vi "Tag Settings Session.vi"(7 "Database Connection":refnum<k7>, 8 "Error In":errorcluster, 10 "DeviceName":string, 11 "Type":enum16{"Set Settings", "Get Settings"}(ring)=enum."Get Settings") -> (0 "Error Out":errorcluster, 3 "Tag Settings":T1(array[cluster]) {"Vmax" min=-10.0 max=10.0 step=1.0; "Vmin" min=-10.0 max=10.0 step=1.0})   [LabVIEW 2019]
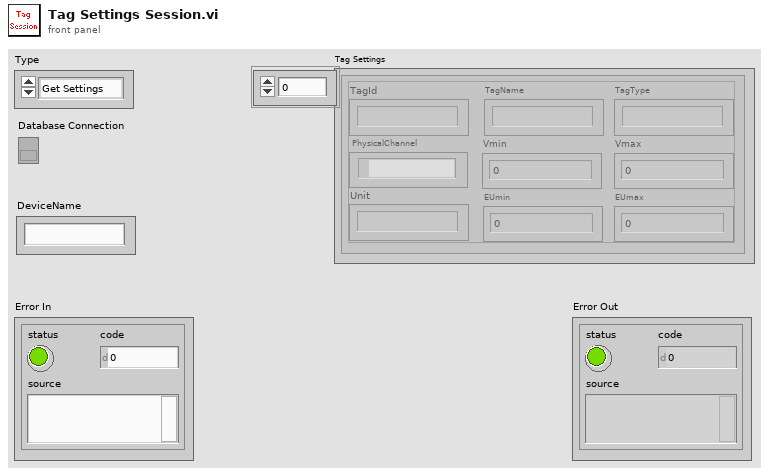
[diagram p1: front panel]
types:
  T1 = cluster{"TagId":string, "TagName":string, "TagType":string, "PhysicalChannel":tag, "Vmin":dbl, "Vmax":dbl, "Unit":string, "EUmin":dbl, "EUmax":dbl}[]
  T2 = cluster{"TagId":string, "TagName":string, "TagType":string, "PhysicalChannel":tag, "Vmin":dbl, "Vmax":dbl, "Unit":string, "EUmin":dbl, "EUmax":dbl}
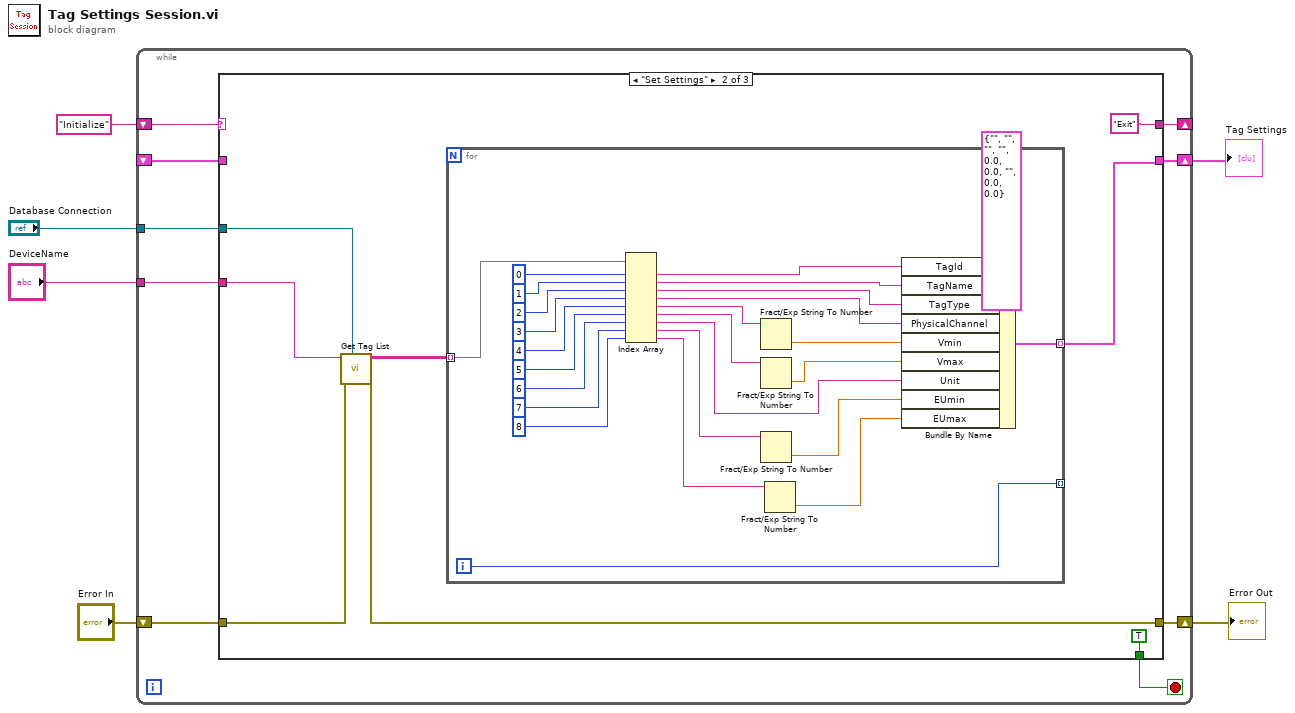
[diagram p0: block diagram]
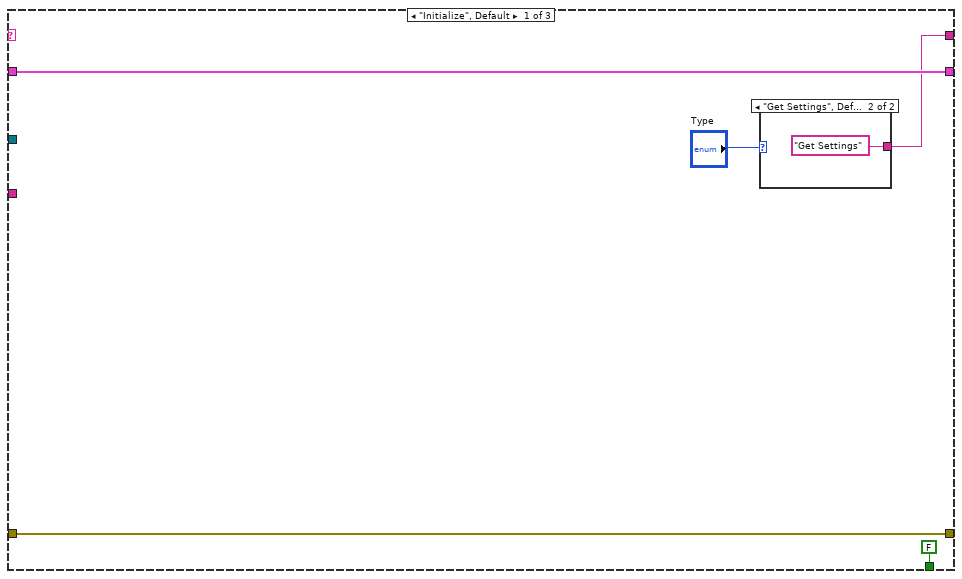
[diagram p2: hidden frame]
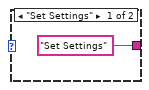
[diagram p3: hidden frame]
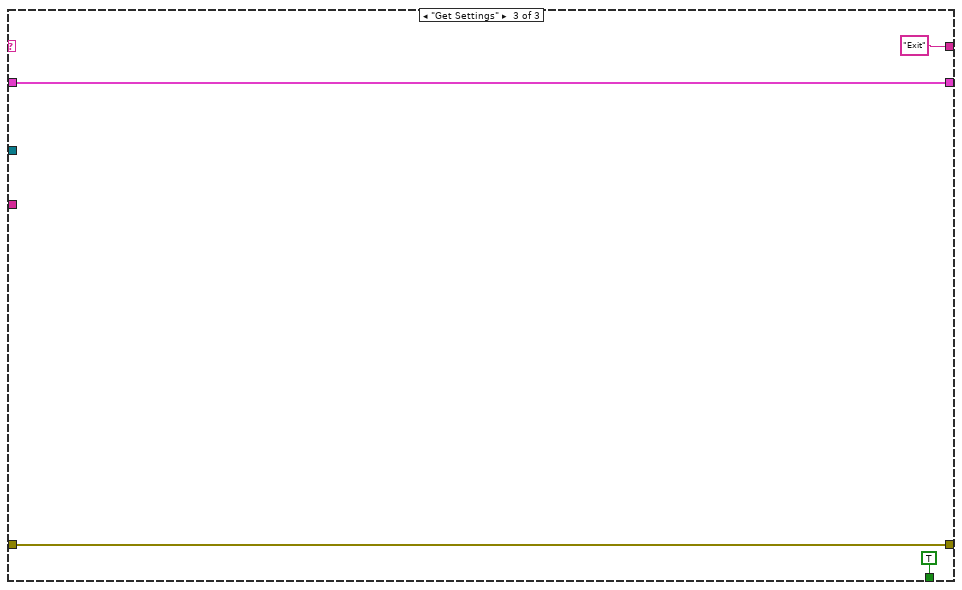
[diagram p4: hidden frame]
diagram:
  n1 = while {
    shift-right: [w10] -> _
    shift-left: "Initialize" ("key") -> [w15]
    shift-right: [w11] -> w3
    shift-left: _ -> [w14]
    shift-right: [w12] -> w4
    shift-left: "Error In" -> [w13]
    tunnel: "Database Connection" -> [w8]
    tunnel: "DeviceName" -> [w7]
    stop <- w9 stop-if-true
    n2 = case shown="\"Set Settings\"" w15 {
      tunnel: w14 -> [w18 _ w57]
      tunnel: w13 -> [w19 w28 w58]
      tunnel: [w19 w27 w58] -> w12
      tunnel: [w18 w23 w57] -> w11
      tunnel: [w16 "Exit" ("key") "Exit" ("key")] -> w10
      tunnel: [FALSE TRUE TRUE] -> w9
      tunnel: w8 -> [_ w26 _]
      tunnel: w7 -> [_ w25 _]
      frame "Initialize", Default {
        n3 = case shown="\"Get Settings\", Default" "Type" {
          tunnel: ["Set Settings" ("key") "Get Settings" ("key")] -> w16
          frame "Set Settings" {
          }
          frame "Get Settings", Default {
          }
        }
      }
      frame "Set Settings" {
        n4 = call "Get Tag List.vi"("Database Connection"=w26, "Error In"=w28, "DeviceName"=w25) -> ("Error Out"=w27:errorcluster, "Tag List"=w24:string[][])  [unwired: 7 in]
        n5 = for {
          tunnel: w24 -> [w55] mode=indexing
          tunnel: [w56] -> w23 mode=indexing
          tunnel: [w31] -> _ mode=indexing
          i -> [w31]
          n6 = Index Array(array=w55, index #1=0 ("index"), index #2=1 ("index"), index #3=2 ("index"), index #4=3 ("index"), index #5=4 ("index"), index #6=5 ("index"), index #7=6 ("index"), index #8=7 ("index"), index #9=8 ("index")) -> (element #1=w53:string, element #2=w44:string, element #3=w43:string, element #4=w42:string, element #5=w41:string, element #6=w38:string, element #7=w37:string, element #8=w36:string, element #9=w34:string)
          n7 = Fract/Exp String To Number(string=w41) -> (number=w40:dbl)  [unwired: 3 in, 1 out]
          n8 = Fract/Exp String To Number(string=w38) -> (number=w39:dbl)  [unwired: 3 in, 1 out]
          n9 = Fract/Exp String To Number(string=w36) -> (number=w35:dbl)  [unwired: 3 in, 1 out]
          n10 = Fract/Exp String To Number(string=w34) -> (number=w33:dbl)  [unwired: 3 in, 1 out]
          n11 = Bundle By Name(cluster=T2 {"TagId"="", "TagName"="", "TagType"="", "PhysicalChannel"="", "Vmin"=0.0, "Vmax"=0.0, "Unit"="", "EUmin"=0.0, "EUmax"=0.0} ("output cluster"), "TagId"=w53, "TagName"=w44, "TagType"=w43, "PhysicalChannel"=w42, "Vmin"=w40, "Vmax"=w39, "Unit"=w37, "EUmin"=w35, "EUmax"=w33) -> (w56:T2)
        }
      }
      frame "Get Settings" {
      }
    }
  }
  "Error Out" <- w4
  "Tag Settings" <- w3
